vi "CAL data.vi"(8 "CAL":T1(array[cluster]), 11 "data out":T3(array[cluster])) -> (3 "CalData":T2(array[cluster]))   [LabVIEW 2011]
uses:
  <vilib>/express/express arith-compare/Formula/XNode/ExpressFormulaBlockNode.xnode
panel:
  out "size(s) 3":i32
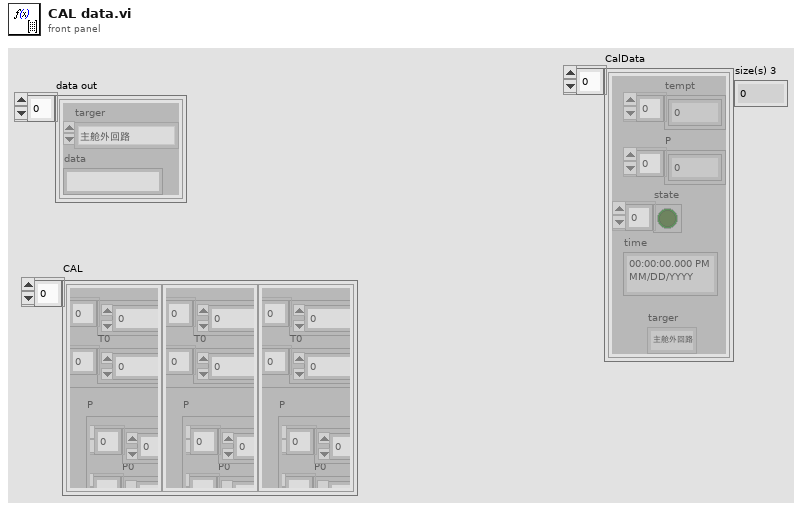
[diagram p1: front panel]
types:
  T1 = cluster{"T":cluster{"TSlop":dbl[], "T0":dbl[]}, "P":cluster{"P0":dbl[], "Pslop":dbl[]}}[]
  T2 = cluster{"tempt":dbl[], "P":dbl[], "state":bool[], "time":timestamp, "targer":enum16{"主舱外回路", "主舱内回路", "实验舱外回路", "实验舱内回路"}}[]
  T3 = cluster{"targer":enum16{"主舱外回路", "主舱内回路", "实验舱外回路", "实验舱内回路"}, "data":string}[]
  T4 = cluster{"tempt":dbl[], "P":dbl[], "state":bool[], "time":timestamp, "targer":enum16{"主舱外回路", "主舱内回路", "实验舱外回路", "实验舱内回路"}}
  T5 = cluster{"T":cluster{"TSlop":dbl[], "T0":dbl[]}, "P":cluster{"P0":dbl[], "Pslop":dbl[]}}
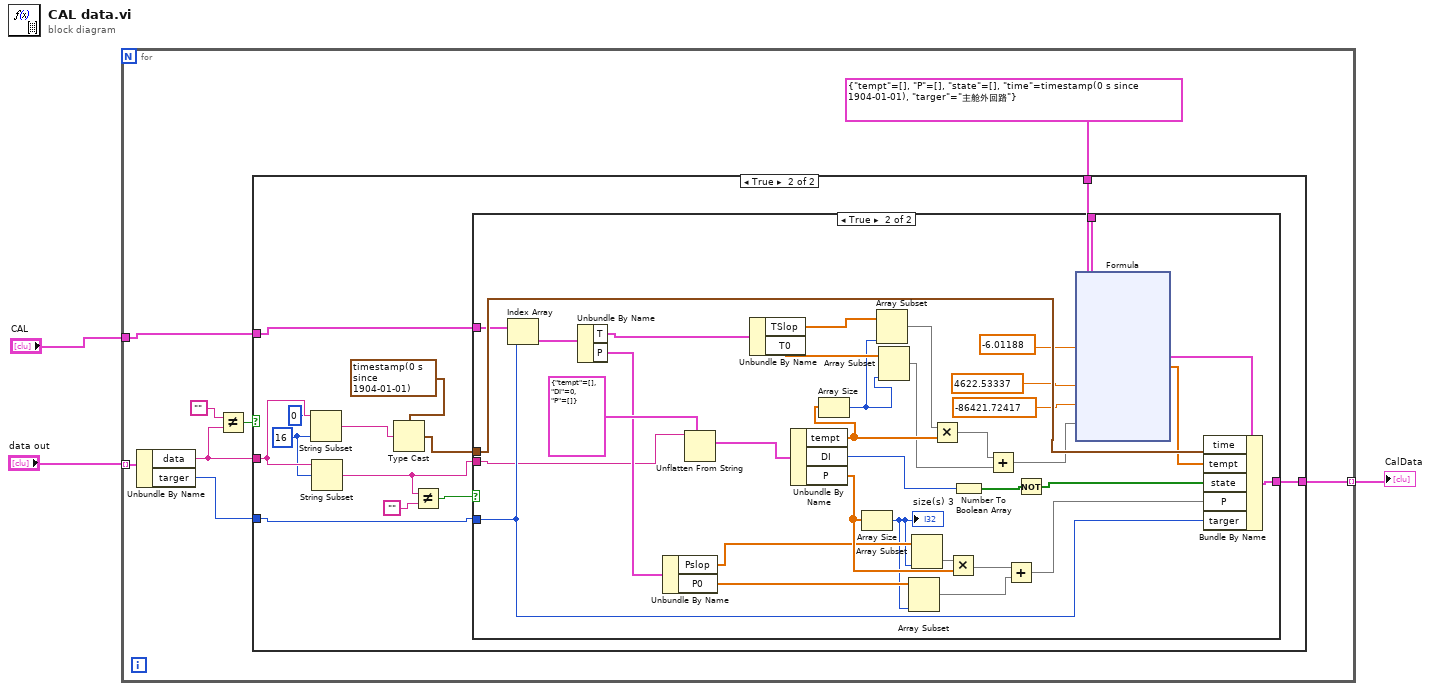
[diagram p0: block diagram]
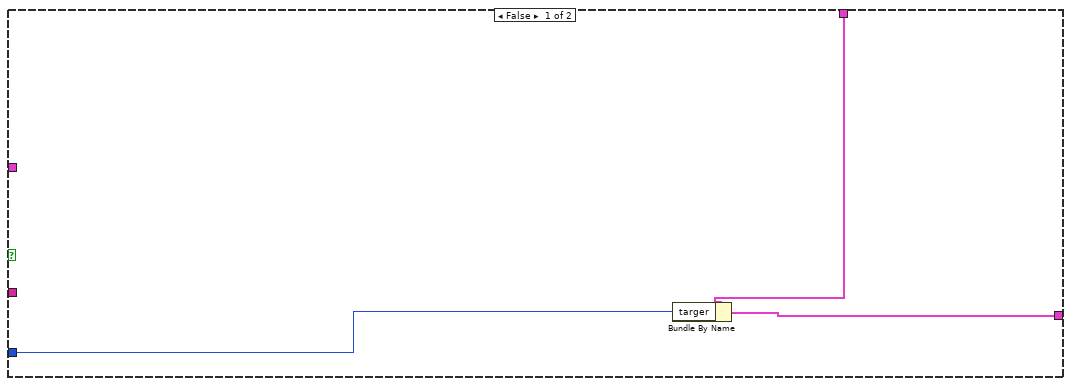
[diagram p2: hidden frame]
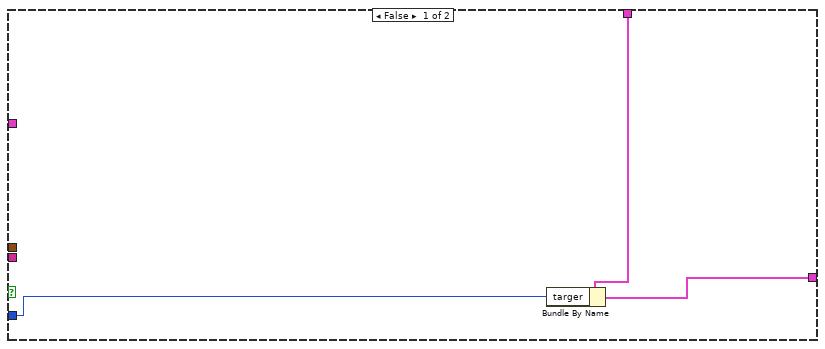
[diagram p3: hidden frame]
diagram:
  n1 = for {
    tunnel: "data out" -> [w11] mode=indexing
    tunnel: [w10] -> w1 mode=indexing
    tunnel: "CAL" -> [w9]
    n2 = Unbundle By Name(w11) -> ("data"=w5:string, "targer"=w8:enum16{"主舱外回路", "主舱内回路", "实验舱外回路", "实验舱内回路"})
    n3 = Not Equal?(x="", y=w5) -> (x != y?=w4:bool)
    n4 = case shown="True" w4 {
      tunnel: w5 -> [_ w21]
      tunnel: [w13 w27] -> w10
      tunnel: w9 -> [_ w26]
      tunnel: w8 -> [w14 w22]
      tunnel: T4 {"tempt"=[], "P"=[], "state"=[], "time"=timestamp(0 s since 1904-01-01), "targer"=enum."主舱外回路"} ("data") -> [w12 w25]
      frame False {
        n5 = Bundle By Name(cluster=w12, "targer"=w14) -> (w13:T4)
      }
      frame True {
        w20 = 16 ("length (rest)")
        n6 = String Subset(string=w21, offset (0)=0, length (rest)=w20) -> (substring=w18:string)
        n7 = String Subset(string=w21, offset (0)=w20) -> (substring=w19:string)  [unwired: 1 in]
        n8 = Type Cast(type=timestamp(0 s since 1904-01-01), x=w18) -> (*(type *) &x=w17:timestamp)
        n9 = Not Equal?(x=w19, y="") -> (x != y?=w23:bool)
        n10 = case shown="True" w23 {
          tunnel: [w30 w57] -> w27
          tunnel: w17 -> [_ w56]
          tunnel: w26 -> [_ w53]
          tunnel: w22 -> [w28 w51]
          tunnel: w25 -> [w29 w50]
          tunnel: w19 -> [_ w49]
          frame False {
            n11 = Bundle By Name(cluster=w29, "targer"=w28) -> (w30:T4)
          }
          frame True {
            n12 = Index Array(array=w53, index=w51) -> (element=w52:T5)
            n13 = Unbundle By Name(w52) -> ("T"=w55:cluster{"TSlop":dbl[], "T0":dbl[]}, "P"=w54:cluster{"P0":dbl[], "Pslop":dbl[]})
            n14 = Unbundle By Name(w54) -> ("Pslop"=w42:dbl[], "P0"=w41:dbl[])
            n15 = Unflatten From String(type=cluster{"tempt":dbl[], "DI":u8, "P":dbl[]} {"tempt"=[], "DI"=0, "P"=[]} ("data"), binary string=w49) -> (value=w63:cluster{"tempt":dbl[], "DI":u8, "P":dbl[]})  [unwired: 3 in, 2 out]
            n16 = Unbundle By Name(w55) -> ("TSlop"=w48:dbl[], "T0"=w44:dbl[])
            n17 = Unbundle By Name(w63) -> ("tempt"=w47:dbl[], "DI"=w60:u8, "P"=w46:dbl[])
            n18 = Array Size(array=w47) -> (size(s)=w43:i32)
            n19 = Array Size(array=w46) -> (size(s)=w40:i32)
            "size(s) 3" <- w40
            n20 = Array Subset(array=w48, length=w43) -> (w45:dbl[])  [unwired: 1 in]
            n21 = Array Subset(array=w44, length=w43) -> (w37:dbl[])  [unwired: 1 in]
            n22 = Array Subset(array=w41, length=w40) -> (w38:dbl[])  [unwired: 1 in]
            n23 = Array Subset(array=w42, length=w40) -> (w39:dbl[])  [unwired: 1 in]
            n24 = Multiply(x=w45, y=w47) -> (x*y=w62:dbl[])
            n25 = Multiply(x=w39, y=w46) -> (x*y=w61:dbl[])
            n26 = Number To Boolean Array(number=w60) -> (Boolean array=w58:bool[])
            n27 = Add(x=w62, y=w37) -> (x+y=w34:dbl[])
            n28 = Add(x=w61, y=w38) -> (x+y=w59:dbl[])
            n29 = Not(x=w58) -> (.not. x?=w36:bool[])
            n30 = xnode "Formula"("a"=-6.01188, "b"=4622.53337, "c"=-86421.72417, "r"=w34) -> ("Result"=w33:dbl[])  [unwired: 1 in, 1 out]
            n31 = Bundle By Name(cluster=w50, "time"=w56, "tempt"=w33, "state"=w36, "P"=w59, "targer"=w51) -> (w57:T4)
          }
        }
      }
    }
  }
  "CalData" <- w1
